vi "TestIntanTimeStamping.vi"() -> ()   [LabVIEW 2012]
panel:
  in  "Digital Trigger Source":tag="/Dev1/PFI1"
  in  "Pulse Duration":dbl=1e-06 format="%.6f"
  in  "Output Terminal":tag="/Dev1/PFI12"
  in  "Counter":tag="Dev1/ctr6"
  in  "Divide By N":dbl=300000.0 format="%.6f"
  in  "Input Terminal":tag="/Dev1/PFI1"
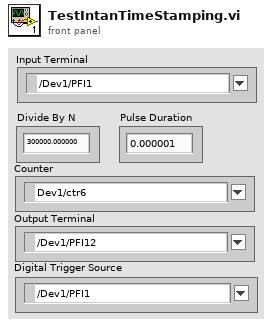
[diagram p1: front panel]
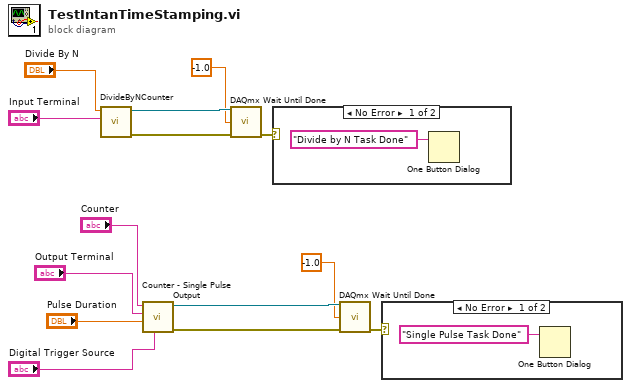
[diagram p0: block diagram]
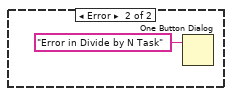
[diagram p2: hidden frame]
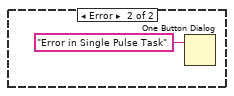
[diagram p3: hidden frame]
diagram:
  n1 = call "DivideByNCounter.vi"("Input Terminal"="Input Terminal", "Divide By N"="Divide By N") -> ("error out"=w5:errorcluster, "task out"=w8:refnum<k21>)  [unwired: 8 in]
  n2 = call "Counter - Single Pulse Output.vi"("Digital Trigger Source"="Digital Trigger Source", "Pulse Duration"="Pulse Duration", "Output Terminal"="Output Terminal", "Counter"="Counter") -> ("error out"=w6:errorcluster, "task out"=w7:refnum<k21>)  [unwired: 6 in]
  n3 = call <vilib>:"DAQmx Wait Until Done.vi"("task/channels in"=w8, "timeout (sec)"=-1.0, "error in"=w5) -> ("error out"=w4:errorcluster)  [unwired: 11 in, 1 out]
  n4 = case shown="No Error" w4 {
    frame No Error {
      n5 = One Button Dialog(message="Divide by N Task Done") -> ()  [unwired: 1 in, 1 out]
    }
    frame Error {
      n6 = One Button Dialog(message="Error in Divide by N Task") -> ()  [unwired: 1 in, 1 out]
    }
  }
  n7 = call <vilib>:"DAQmx Wait Until Done.vi"("task/channels in"=w7, "timeout (sec)"=-1.0, "error in"=w6) -> ("error out"=w3:errorcluster)  [unwired: 11 in, 1 out]
  n8 = case shown="No Error" w3 {
    frame No Error {
      n9 = One Button Dialog(message="Single Pulse Task Done") -> ()  [unwired: 1 in, 1 out]
    }
    frame Error {
      n10 = One Button Dialog(message="Error in Single Pulse Task") -> ()  [unwired: 1 in, 1 out]
    }
  }
